vi "UsrProfiles-Delete profile.vi"   [LabVIEW 2020]
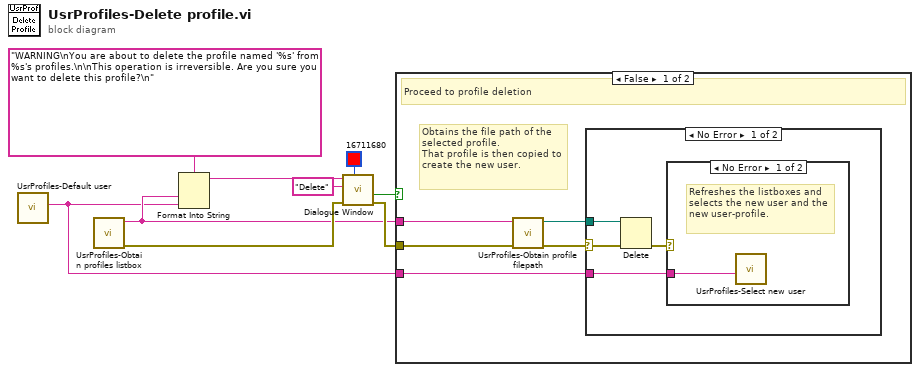
[diagram p0: block diagram]
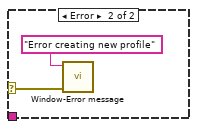
[diagram p2: hidden frame]
diagram:
  n1 = call "UsrProfiles-Default user.vi"() -> ("Selected user's name"=w2:string)  [unwired: 9 in, 2 out]
  n2 = call "UsrProfiles-Obtain profiles listbox.vi"() -> ("error out"=w4:errorcluster, "Selected profile's name"=w3:string)  [unwired: 8 in, 2 out]
  n3 = Format Into String(format string="WARNING\nYou are about to delete the profile named '%s' from %s's profiles.\n\nThis operation is irreversible. Are you sure you want to delete this profile?\n" ("Message string"), w3, w2) -> (resulting string=w8:string)  [unwired: 2 in, 1 out]
  n4 = call "Dialogue Window.vi"("Colour"=u32 16711680, "error in (no error)"=w4, "Caption-Right button (OK)"="Delete", "Message string"=w8) -> ("error out"=w5:errorcluster, "Cancelled (Left button pressed)"=w6:bool)  [unwired: 5 in, 1 out]
  n5 = case shown="False" w6 {
    tunnel: w3 -> [w14 _]
    tunnel: w5 -> [w13 _]
    tunnel: w2 -> [w11 _]
    frame False {
      # "Obtains the file path of the selected profile.\nThat profile is then copied to create the new user."
      # "Proceed to profile deletion"
      n6 = call "UsrProfiles-Obtain profile filepath.vi"("error in"=w13, "Profile name"=w14) -> ("error out"=w12:errorcluster, "Profile filepath"=w10:path)  [unwired: 8 in]
      n7 = case shown="No Error" w12 {
        selector: w12 -> [w16 _]
        tunnel: w11 -> [w15 _]
        tunnel: w10 -> [w18 _]
        frame No Error {
          n8 = Delete(path (use dialog)=w18, error in=w16) -> (error out=w17:errorcluster)  [unwired: 3 in, 2 out]
          n9 = case shown="No Error" w17 {
            selector: w17 -> [_ w20]
            tunnel: w15 -> [w19 _]
            frame No Error {
              # "Refreshes the listboxes and selects the new user and the new user-profile."
              n10 = call "UsrProfiles-Select new user.vi"("New user name"=w19) -> ()  [unwired: 11 in]
            }
            frame Error {
              n11 = call "Window-Error message.vi"("error in (no error)"=w20, "Message"="Error creating new profile") -> ()  [unwired: 9 in, 1 out]
            }
          }
        }
        frame Error {
        }
      }
    }
    frame True {
      # "Cancelled"
    }
  }
